vi "Read TDMS XYN.vi"(8 "error in (no error)":errorcluster, 9 "Channels":cluster{"X":string, "Y":string, "N":string}, 11 "File or Folder Path":path=path "C:/") -> (0 "error out":errorcluster, 1 "N []":dbl[](array[numeric]), 2 "Y vs X []":cluster{dbl[], dbl[]}[](graph))   [LabVIEW 2019, in "Data.TDMS.lvclass"]
uses:
  Data.TDMS.lvclass
panel:
  out "Path":path
  in  "length":i32=1
  out "counter":i32
  in  "offset":i32
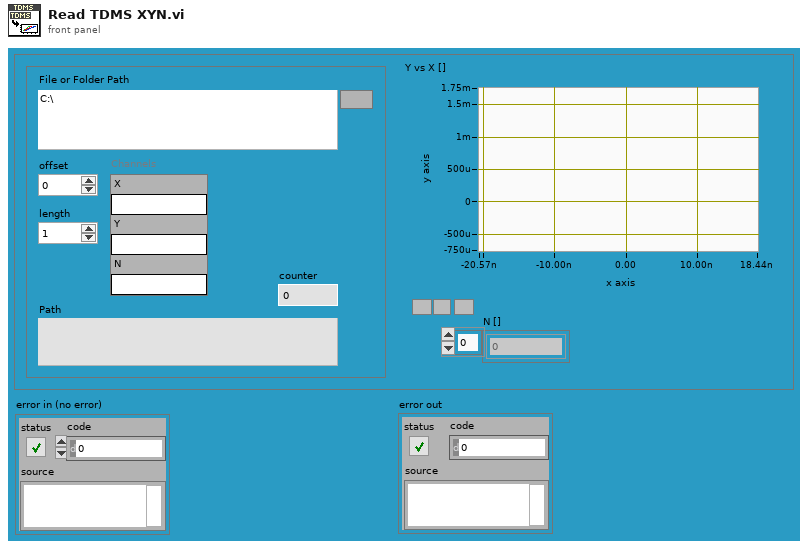
[diagram p1: front panel]
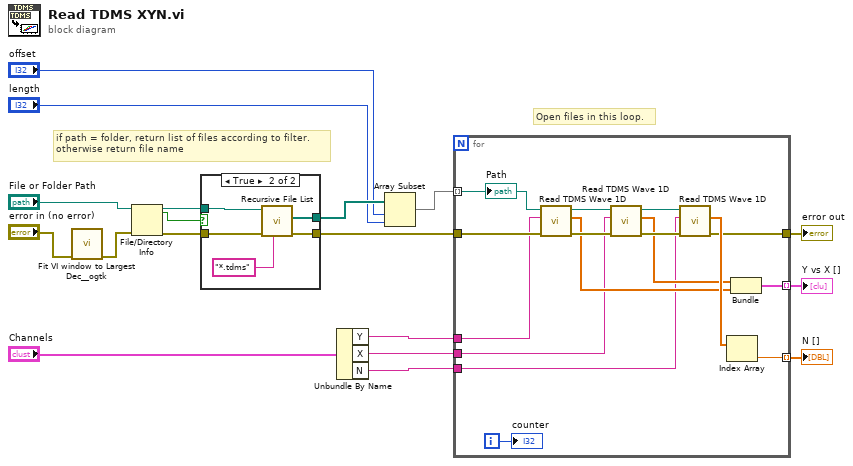
[diagram p0: block diagram]
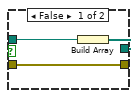
[diagram p2: hidden frame]
diagram:
  # "Open files in this loop."
  # "if path = folder, return list of files according to filter.\notherwise return file name"
  n1 = call "Fit VI window to Largest Dec__ogtk.vi"("error in (no error)"="error in (no error)") -> ("error out"=w9:errorcluster)  [unwired: 5 in, 1 out]
  n2 = File/Directory Info(path="File or Folder Path", error in=w9) -> (path out=w11:path, directory=w13:bool, error out=w12:errorcluster)  [unwired: 4 out]
  n3 = case shown="True" w13 {
    tunnel: [w21 w25] -> w18
    tunnel: w11 -> [w20 w26]
    tunnel: w12 -> [w19 w24]
    tunnel: [w19 w23] -> w14
    frame False {
      n4 = Build Array(w20) -> (w21:path[])
    }
    frame True {
      n5 = call <vilib>:"Recursive File List.vi"("pattern"="*.tdms", "error in (no error)"=w24, "Folder Path"=w26) -> ("error out"=w23:errorcluster, "All Files in Dir"=w25:path[])  [unwired: 4 in, 3 out]
    }
  }
  n6 = Unbundle By Name("Channels") -> ("Y"=w8:string, "X"=w7:string, "N"=w6:string)
  n7 = Array Subset(array=w18, index="offset", length="length") -> (w2:path[])
  n8 = for {
    tunnel: w2 -> [w30] mode=indexing
    tunnel: [w41] -> w1 mode=indexing
    tunnel: w14 -> [w40]
    tunnel: [w34] -> w4 mode=indexing
    tunnel: [w33] -> w5
    tunnel: w8 -> [w29]
    tunnel: w7 -> [w27]
    tunnel: w6 -> [w28]
    i -> [w42]
    n9 = call "Read TDMS Wave 1D.vi"("error in (no error)"=w40, "channel name(s) in"=w29, "path"=w30) -> ("error out"=w39:errorcluster, "data"=w31:dbl[], "file path out"=w38:path)  [unwired: 6 in]
    n10 = call "Read TDMS Wave 1D.vi"("error in (no error)"=w39, "channel name(s) in"=w27, "path"=w38) -> ("error out"=w37:errorcluster, "data"=w32:dbl[], "file path out"=w36:path)  [unwired: 6 in]
    n11 = call "Read TDMS Wave 1D.vi"("error in (no error)"=w37, "channel name(s) in"=w28, "path"=w36) -> ("error out"=w33:errorcluster, "data"=w35:dbl[])  [unwired: 6 in, 1 out]
    n12 = Index Array(array=w35) -> (element=w34:dbl)  [unwired: 1 in]
    n13 = Bundle("data"=w32, "data"=w31) -> (w41:cluster{"data":dbl[], "data":dbl[]})  [unwired: 1 in]
    "counter" <- w42
    "Path" <- w30
  }
  "error out" <- w5
  "Y vs X []" <- w1
  "N []" <- w4
